vi "Arrange VIWin - Get FP Controls Rows.vi"(0 "controls":T1[](array[typedef])) -> (4 "top row":T1[](array[typedef]), 6 "middle rows":T1[](array[typedef]), 8 "bottom row":T1[](array[typedef]))   [LabVIEW 2020, in "Arrange VI Window.lvlib"]
uses:
  Arrange VI Window.lvlib
  Arrange VIWin - FP Control Info.ctl
  <vilib>/Utility/miscctls.llb/LVRectTypeDef.ctl
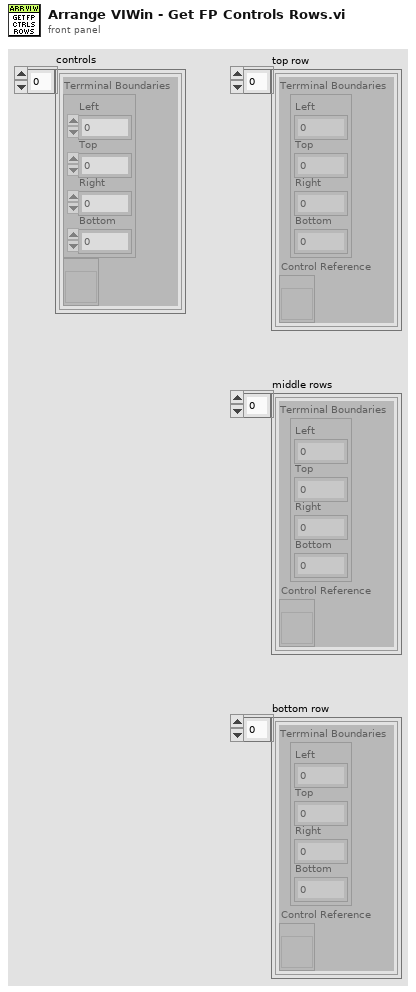
[diagram p1: front panel]
types:
  T1 = typedef "Arrange VI Window.lvlib/Arrange VIWin - FP Control Info.ctl" = cluster{"Terrminal Boundaries":T2, "Control Reference":refnum<vi>}
  T2 = typedef "LVRectTypeDef.ctl" = cluster{"Left":i16, "Top":i16, "Right":i16, "Bottom":i16}
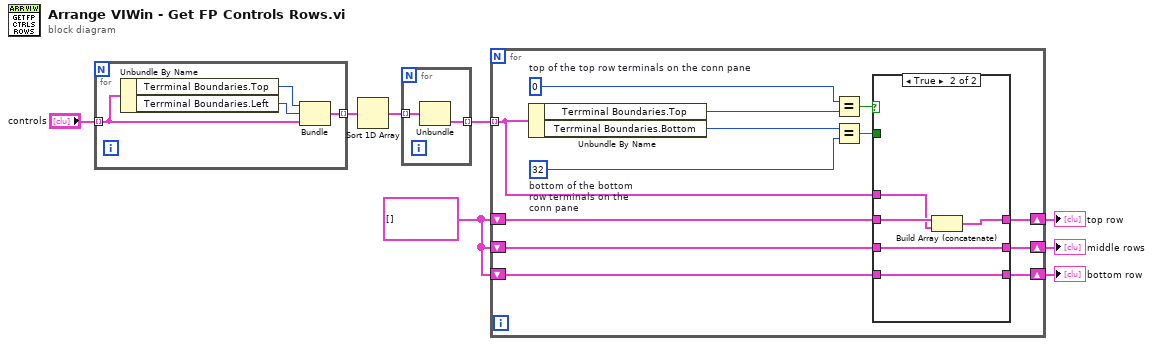
[diagram p0: block diagram]
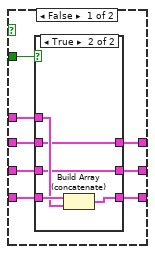
[diagram p2: hidden frame]
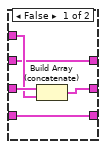
[diagram p3: hidden frame]
diagram:
  w6 = T1[] [] ("sorted array of control info")
  n1 = for {
    tunnel: "controls" -> [w11] mode=indexing
    tunnel: [w10] -> w3 mode=indexing
    n2 = Unbundle By Name(w11) -> ("Terrminal Boundaries.Top"=w12:i16, "Terrminal Boundaries.Left"=w9:i16)
    n3 = Bundle("Top"=w12, "Left"=w9, w11) -> (w10:cluster{"Top":i16, "Left":i16, T1})  [unwired: 1 in]
  }
  n4 = Sort 1D Array(array=w3) -> (sorted array=w2:cluster{"Top":i16, "Left":i16, T1}[])
  n5 = for {
    tunnel: w2 -> [w14] mode=indexing
    tunnel: [w13] -> w1 mode=indexing
    n6 = Unbundle(w14) -> (w13:T1)  [unwired: 2 out]
  }
  n7 = for {
    shift-right: [w22] -> w8
    shift-left: w6 -> [w26]
    tunnel: w1 -> [w24] mode=indexing
    shift-right: [w21] -> w7
    shift-left: w6 -> [w20]
    shift-right: [w16] -> w5
    shift-left: w6 -> [w17]
    w19 = i16 0  # top of the top row terminals on the conn pane
    w27 = i16 32  # bottom of the bottom row terminals on the conn pane
    n8 = Unbundle By Name(w24) -> ("Terrminal Boundaries.Top"=w18:i16, "Terrminal Boundaries.Bottom"=w23:i16)
    n9 = Equal?(x=w19, y=w18) -> (x = y?=w15:bool)
    n10 = Equal?(x=w23, y=w27) -> (x = y?=w25:bool)
    n11 = case shown="True" w15 {
      tunnel: w26 -> [w35 w47]
      tunnel: w25 -> [w34 _]
      tunnel: w24 -> [w33 w49]
      tunnel: [w32 w47] -> w22
      tunnel: [w31 w46] -> w21
      tunnel: w20 -> [w30 w46]
      tunnel: w17 -> [w29 w50]
      tunnel: [w28 w48] -> w16
      frame False {
        n12 = case shown="True" w34 {
          tunnel: [w40 w45] -> w32
          tunnel: w35 -> [w40 w44]
          tunnel: w33 -> [w37 w43]
          tunnel: [w38 w42] -> w31
          tunnel: w30 -> [w39 w42]
          tunnel: w29 -> [w36 w41]
          tunnel: [w36 w41] -> w28
          frame False {
            n13 = Build Array (concatenate)(w39, w37) -> (w38:T1[])
          }
          frame True {
            n14 = Build Array (concatenate)(w44, w43) -> (w45:T1[])
          }
        }
      }
      frame True {
        n15 = Build Array (concatenate)(w50, w49) -> (w48:T1[])
      }
    }
  }
  "bottom row" <- w8
  "middle rows" <- w7
  "top row" <- w5
